vi "AlazarReadRegister.vi"(4 "error in (no error)":errorcluster, 5 "Password":u32, 6 "Offset":u32, 7 "Board Handle":u64) -> (0 "error out":errorcluster, 1 "Return Code":u32, 2 "Value Out":u32, 3 "Board Handle Out":u64)   [LabVIEW 2009]
uses:
  ATSApi.dll
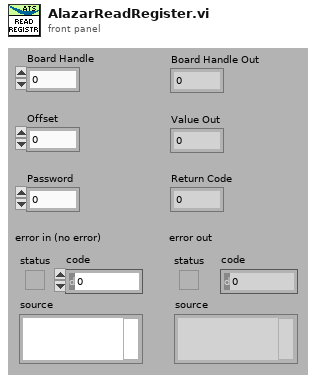
[diagram p1: front panel]
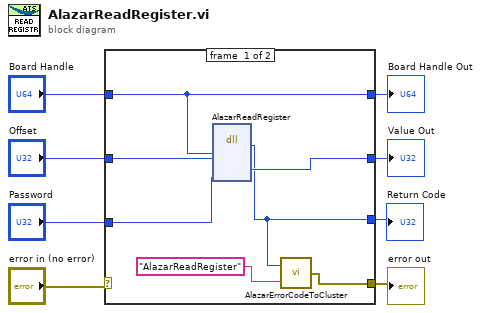
[diagram p0: block diagram]
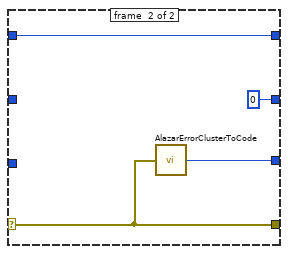
[diagram p2: hidden frame]
diagram:
  n1 = case shown="No Error" "error in (no error)" {
    selector: "error in (no error)" -> [_ w17]
    tunnel: [w9 w17] -> w7
    tunnel: [w12 u32 0] -> w6
    tunnel: [w15 w18] -> w5
    tunnel: "Board Handle" -> [w15 w18]
    tunnel: [w11 w16] -> w3
    tunnel: "Offset" -> [w14 _]
    tunnel: "Password" -> [w13 _]
    frame #0 {
      n2 = dll-call lib="ATSApi.dll" fn="AlazarReadRegister"("handle"=w15, "offset"=w14, "password"=w13) -> ("return type"=w11:u32, "retVal"=w12:u32)  [unwired: 7 in, 2 out]
      n3 = call "AlazarErrorCodeToCluster.vi"("Message"="AlazarReadRegister", "Error Code"=w11) -> ("error out"=w9:errorcluster)
    }
    frame #1 {
      n4 = call "AlazarErrorClusterToCode.vi"("error in (no error)"=w17) -> ("Error Code"=w16:u32)
    }
  }
  "Board Handle Out" <- w5
  "Value Out" <- w6
  "error out" <- w7
  "Return Code" <- w3
